vi "Configure.vi"(8 "error in (no error)":errorcluster, 9 "Path":path, 10 "Interactive?":bool, 11 "Text Report In":refnum<class "Text Report.lvclass">) -> (0 "error out":errorcluster, 3 "Text Report Out":refnum<class "Text Report.lvclass">)   [LabVIEW 2020, in "Text Report.lvclass"]
uses:
  Text Report.lvclass
  Text Report.lvclass/Text Report.ctl
  <vilib>/Utility/sysdir.llb/Get System Directory.vi
  <vilib>/Utility/libraryn.llb/Create Directory Recursive.vi
  User Interface/Configuration Manager/Configuration Manager.lvclass
  User Interface/Support/Paths.lvlib
panel:
  in  "Cancel":bool
  in  "Commit":bool
  in  "Open New Reports":bool
  in  "Report Path":path
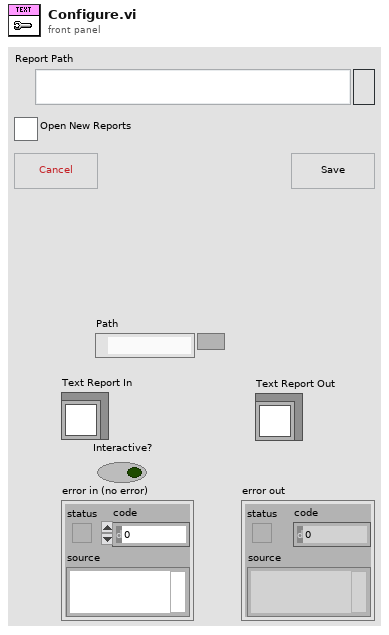
[diagram p1: front panel]
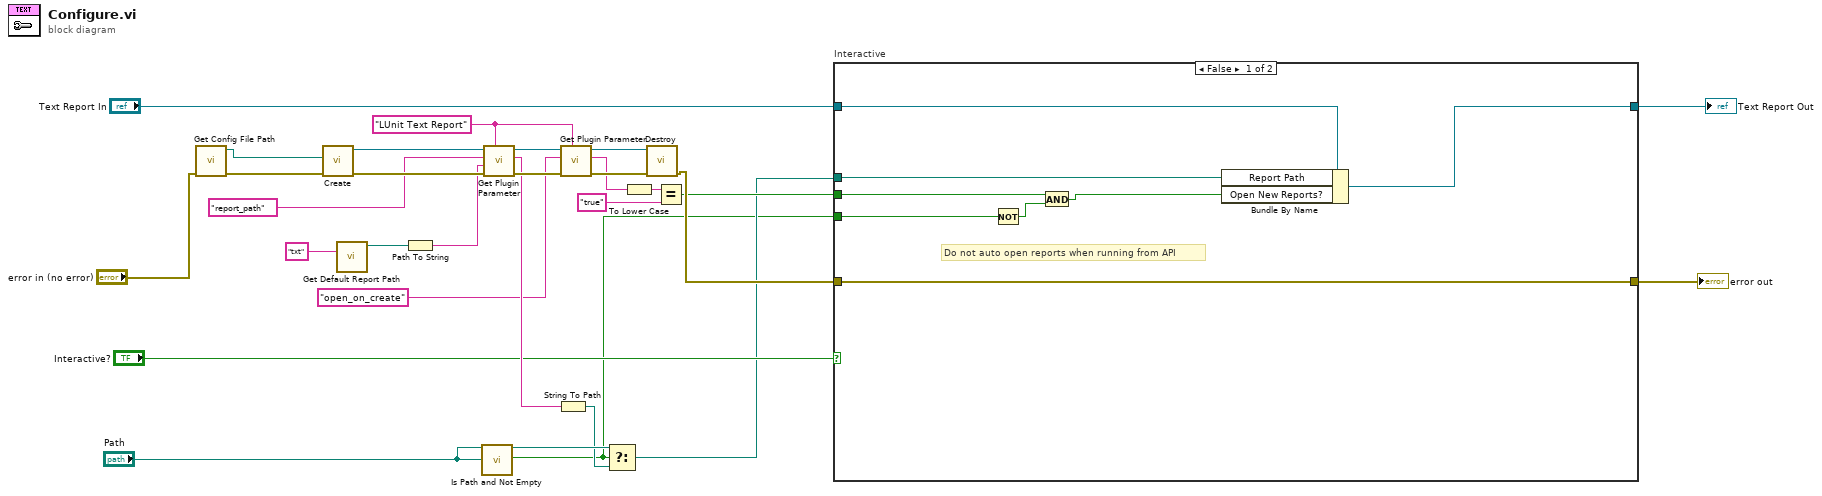
[diagram p0: block diagram]
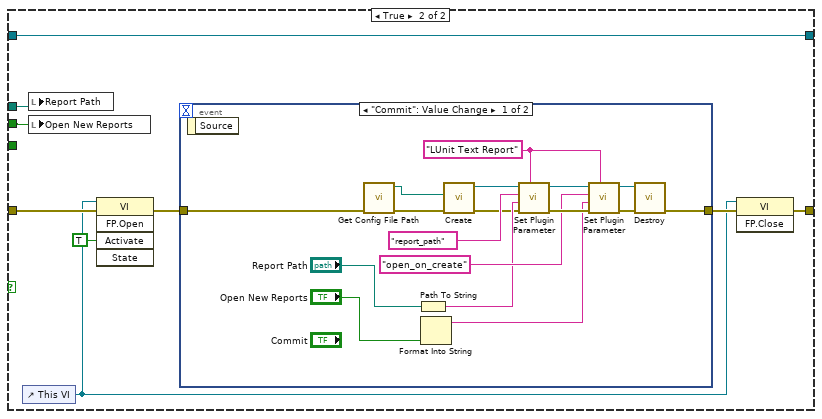
[diagram p2: hidden frame]
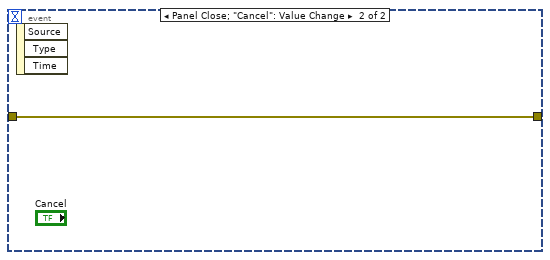
[diagram p3: hidden frame]
diagram:
  w15 = "LUnit Text Report"
  n1 = call "Get Config File Path.vi"("error in (no error)"="error in (no error)") -> ("error out"=w28:errorcluster, "Config Directory"=w27:path)  [unwired: 9 in]
  n2 = call "Create.vi"("error in (no error)"=w28, "configuration file path"=w27) -> ("error out"=w25:errorcluster, "Configuration Manager out"=w29:refnum<class "Configuration Manager.lvclass">)  [unwired: 8 in]
  n3 = call "Get Default Report Path.vi"("File Extension"="txt") -> ("Default Report Path"=w7:path)  [unwired: 9 in, 1 out]
  n4 = Path To String(path=w7) -> (string=w6:string)
  n5 = call <vilib>:"Is Path and Not Empty.vi"("path"="Path") -> ("Is Path and Not Empty?"=w1:bool)  [unwired: 4 in]
  n6 = call "Get Plugin Parameter.vi"("Plugin"=w15, "error in (no error)"=w25, "Default Value"=w6, "Name"="report_path", "Configuration Manager in"=w29) -> ("error out"=w26:errorcluster, "Value"=w23:string, "Configuration Manager out"=w21:refnum<class "Configuration Manager.lvclass">)  [unwired: 4 in]
  n7 = String To Path(string=w23) -> (path=w4:path)
  n8 = call "Get Plugin Parameter.vi"("Plugin"=w15, "error in (no error)"=w26, "Name"="open_on_create", "Configuration Manager in"=w21) -> ("error out"=w22:errorcluster, "Value"=w18:string, "Configuration Manager out"=w20:refnum<class "Configuration Manager.lvclass">)  [unwired: 5 in]
  n9 = Select(t="Path", s=w1, f=w4) -> (s? t:f=w2:path)
  n10 = To Lower Case(string=w18) -> (all lower case string=w17:string)
  n11 = call "Destroy.vi"("error in (no error)"=w22, "Configuration Manager In"=w20) -> ("error out"=w13:errorcluster)  [unwired: 9 in]
  n12 = Equal?(x=w17, y="true") -> (x = y?=w3:bool)
  n13 = case "Interactive" shown="False" "Interactive?" {
    tunnel: w13 -> [w37 w44]
    tunnel: [w37 w42] -> w12
    tunnel: "Text Report In" -> [w36 w40]
    tunnel: [w35 w40] -> w9
    tunnel: w3 -> [w34 w39]
    tunnel: w2 -> [w33 w38]
    tunnel: w1 -> [w30 _]
    frame False {
      # "Do not auto open reports when running from API"
      n14 = Not(x=w30) -> (.not. x?=w31:bool)
      n15 = And(x=w34, y=w31) -> (x .and. y?=w32:bool)
      n16 = Bundle By Name(cluster=w36, "Report Path"=w33, "Open New Reports?"=w32) -> (w35:refnum<class "Text Report.lvclass">)
    }
    frame True {
      n17 = control-ref of="This VI"() -> (w41:refnum<vi>)
      n18 = local write "Report Path"(w38) -> ()
      n19 = local write "Open New Reports"(w39) -> ()
      n20 = invoke class="VI" method="FP.Open"(reference=w41, error in=w44, "Activate"=TRUE ("Activate?")) -> (error out=w45:errorcluster)  [unwired: 2 in, 4 out]
      n21 = event shown="[0] \"Commit\": Value Change" {
        selector: _ -> [_ _]
        dyn-events: _ -> [_ _]
        timeout: _ -> [_ _]
        tunnel: w45 -> [w61 w64]
        tunnel: [w60 w64] -> w43
        event "Commit": Value Change {
          w59 = "LUnit Text Report"
          n22 = event-data() -> ()  [unwired: 1 in, 1 out]
          n23 = call "Get Config File Path.vi"("error in (no error)"=w61) -> ("error out"=w52:errorcluster, "Config Directory"=w51:path)  [unwired: 9 in]
          n24 = Path To String(path="Report Path") -> (string=w54:string)
          n25 = Format Into String("Open New Reports") -> (resulting string=w53:string)  [unwired: 3 in, 1 out]
          n26 = call "Create.vi"("error in (no error)"=w52, "configuration file path"=w51) -> ("error out"=w49:errorcluster, "Configuration Manager out"=w50:refnum<class "Configuration Manager.lvclass">)  [unwired: 8 in]
          n27 = call "Set Plugin Parameter.vi"("Plugin"=w59, "error in (no error)"=w49, "Value"=w54, "Name"="report_path", "Configuration Manager in"=w50) -> ("error out"=w57:errorcluster, "Configuration Manager out"=w58:refnum<class "Configuration Manager.lvclass">)  [unwired: 5 in]
          n28 = call "Set Plugin Parameter.vi"("Plugin"=w59, "error in (no error)"=w57, "Value"=w53, "Name"="open_on_create", "Configuration Manager in"=w58) -> ("error out"=w47:errorcluster, "Configuration Manager out"=w48:refnum<class "Configuration Manager.lvclass">)  [unwired: 5 in]
          n29 = call "Destroy.vi"("error in (no error)"=w47, "Configuration Manager In"=w48) -> ("error out"=w60:errorcluster)  [unwired: 9 in]
        }
        event Panel Close; "Cancel": Value Change {
          n30 = event-data() -> ()  [unwired: 1 in, 3 out]
        }
      }
      n31 = invoke class="VI" method="FP.Close"(reference=w41, error in=w43) -> (error out=w42:errorcluster)  [unwired: 1 in, 2 out]
    }
  }
  "error out" <- w12
  "Text Report Out" <- w9
